vi "CRYDigital IO Setting.vi"(6 "No.VI":i32, 10 "Message Cluster":T1={"Name"="Default", "Type"=0, "Command Msg"="<Enter message or command here>", "Flags"=0, "Dialog?"=FALSE, "Numeric?"=FALSE, "Wait?"=FALSE, "Pause [ms]"=0, "pattern"=0, "Address"="", "Operation"=0, "bytes"=0, "Line selected"=0, "RS232 Func"=0, "Serial Ctrl lines"=0, "Interf #"=0, "GPIB func"=0, "GPIB cmd"=0, "GPIB rem en"=FALSE, "GPIB term"=0, "Curves generated"=[], "Units"={"unit"="", "dB ref"=0.0, "axis"=0, "data"=0, "Common dB ref."=1}, "Axis"=0, "Default Value"=0.0, "Message Tilte"="", "Port #"=0, "Print Unit"="", "Text Format"={"Size"=0, "Plain"=FALSE, "Bold"=FALSE, "Italic"=FALSE, "Underline"=FALSE, "Strikethrough"=FALSE, "Color"=0, "Font"=""}, "Help"="", "Tab Value"=enum."Setting", "pattern 2"=0, "Line selected 2"=0, "H_Bits"=[], "G_Bits"=[]} {"pattern 2" format="%.0b"; "Units"."Common dB ref." items=["dB", "dBSPL", "dBPa", "dBV", "dBm", "dBu", "dBFS"]; "Units"."dB ref" format="%.2f"; "pattern" format="%.0b"; "Flags" items=["Pass", "Fail"]}) -> (0 "Result":bool, 3 "Message Cluster Out":T1={"Name"="Default", "Type"=0, "Command Msg"="<Enter message or command here>", "Flags"=0, "Dialog?"=FALSE, "Numeric?"=FALSE, "Wait?"=FALSE, "Pause [ms]"=0, "pattern"=0, "Address"="", "Operation"=0, "bytes"=0, "Line selected"=0, "RS232 Func"=0, "Serial Ctrl lines"=0, "Interf #"=0, "GPIB func"=0, "GPIB cmd"=0, "GPIB rem en"=FALSE, "GPIB term"=0, "Curves generated"=[], "Units"={"unit"="", "dB ref"=0.0, "axis"=0, "data"=0, "Common dB ref."=1}, "Axis"=0, "Default Value"=0.0, "Message Tilte"="", "Port #"=0, "Print Unit"="", "Text Format"={"Size"=0, "Plain"=FALSE, "Bold"=FALSE, "Italic"=FALSE, "Underline"=FALSE, "Strikethrough"=FALSE, "Color"=0, "Font"=""}, "Help"="", "Tab Value"=enum."Setting", "pattern 2"=0, "Line selected 2"=0, "H_Bits"=[], "G_Bits"=[]} {"pattern 2" format="%.0b"; "Units"."Common dB ref." items=["dB", "dBSPL", "dBPa", "dBV", "dBm", "dBu", "dBFS"]; "Units"."dB ref" format="%.2f"; "pattern" format="%.0b"; "Flags" items=["Pass", "Fail"]})   [LabVIEW 2013]
uses:
  Typedef Control/CRYMessages Cluster.ctl
panel:
  out "H Selected":bool[](array[boolean])
  out "G Selected":bool[](array[boolean])
  out "Total_Comment":string
  out "True_Comment":string
  out "False_Comment":string
  out "G_Bits Out":T2(array[cluster])
  out "H_Bits Out":T2(array[cluster])
  out "Invert True":bool=TRUE caption="Invert"
  out "Invert False":bool=TRUE caption="Invert"
  in  "Setting Tab":enum32{"Port G", "Port H"}(tab)
  in  "G_Invert 2":bool=TRUE caption="Invert"
  in  "G_Invert 0":bool=TRUE caption="Invert"
  in  "G_Bit 4":i32[](listbox) caption="Bit 4"
  in  "G_Bit 0":i32[](listbox) caption="Bit 0"
  in  "G_Bit 1":i32[](listbox) caption="Bit 1"
  in  "G_Bit 3":i32[](listbox) caption="Bit 3"
  in  "G_Bit 5":i32[](listbox) caption="Bit 5"
  in  "G_Bit 7":i32[](listbox) caption="Bit 7"
  in  "G_Invert 1":bool=TRUE caption="Invert"
  in  "G_All 0":bool=TRUE caption="All"
  in  "G_All 1":bool=TRUE caption="All"
  in  "G_All 2":bool=TRUE caption="All"
  in  "G_All 3":bool=TRUE caption="All"
  in  "G_All 4":bool=TRUE caption="All"
  in  "G_All 5":bool=TRUE caption="All"
  in  "G_All 6":bool=TRUE caption="All"
  in  "G_All 7":bool=TRUE caption="All"
  in  "G_Invert 3":bool=TRUE caption="Invert"
  in  "G_Bit 2":i32[](listbox) caption="Bit 2"
  in  "G_Invert 4":bool=TRUE caption="Invert"
  in  "G_Invert 5":bool=TRUE caption="Invert"
  in  "G_Invert 6":bool=TRUE caption="Invert"
  in  "G_Bit 6":i32[](listbox) caption="Bit 6"
  in  "G_Invert 7":bool=TRUE caption="Invert"
  in  "H_All 0":bool=TRUE caption="All"
  in  "H_All 1":bool=TRUE caption="All"
  in  "H_All 2":bool=TRUE caption="All"
  in  "H_All 3":bool=TRUE caption="All"
  in  "H_All 4":bool=TRUE caption="All"
  in  "H_All 5":bool=TRUE caption="All"
  in  "H_All 6":bool=TRUE caption="All"
  in  "H_All 7":bool=TRUE caption="All"
  in  "H_Bit 7":i32[](listbox) caption="Bit 7"
  in  "H_Invert 7":bool=TRUE caption="Invert"
  in  "H_Bit 6":i32[](listbox) caption="Bit 6"
  in  "H_Invert 6":bool=TRUE caption="Invert"
  in  "H_Bit 5":i32[](listbox) caption="Bit 5"
  in  "H_Invert 5":bool=TRUE caption="Invert"
  in  "H_Bit 4":i32[](listbox) caption="Bit 4"
  in  "H_Invert 4":bool=TRUE caption="Invert"
  in  "H_Bit 3":i32[](listbox) caption="Bit 3"
  in  "H_Invert 3":bool=TRUE caption="Invert"
  in  "H_Bit 2":i32[](listbox) caption="Bit 2"
  in  "H_Invert 2":bool=TRUE caption="Invert"
  in  "H_Bit 1":i32[](listbox) caption="Bit 1"
  in  "H_Invert 1":bool=TRUE caption="Invert"
  in  "H_Bit 0":i32[](listbox) caption="Bit 0"
  in  "H_Invert 0":bool=TRUE caption="Invert"
  in  "Cancel":bool
  in  "OK":bool
  # "Ture = On     False = Off"
  # "Ture = Off     False = On"
  # "The results are \"Boolean And\" of items selected."
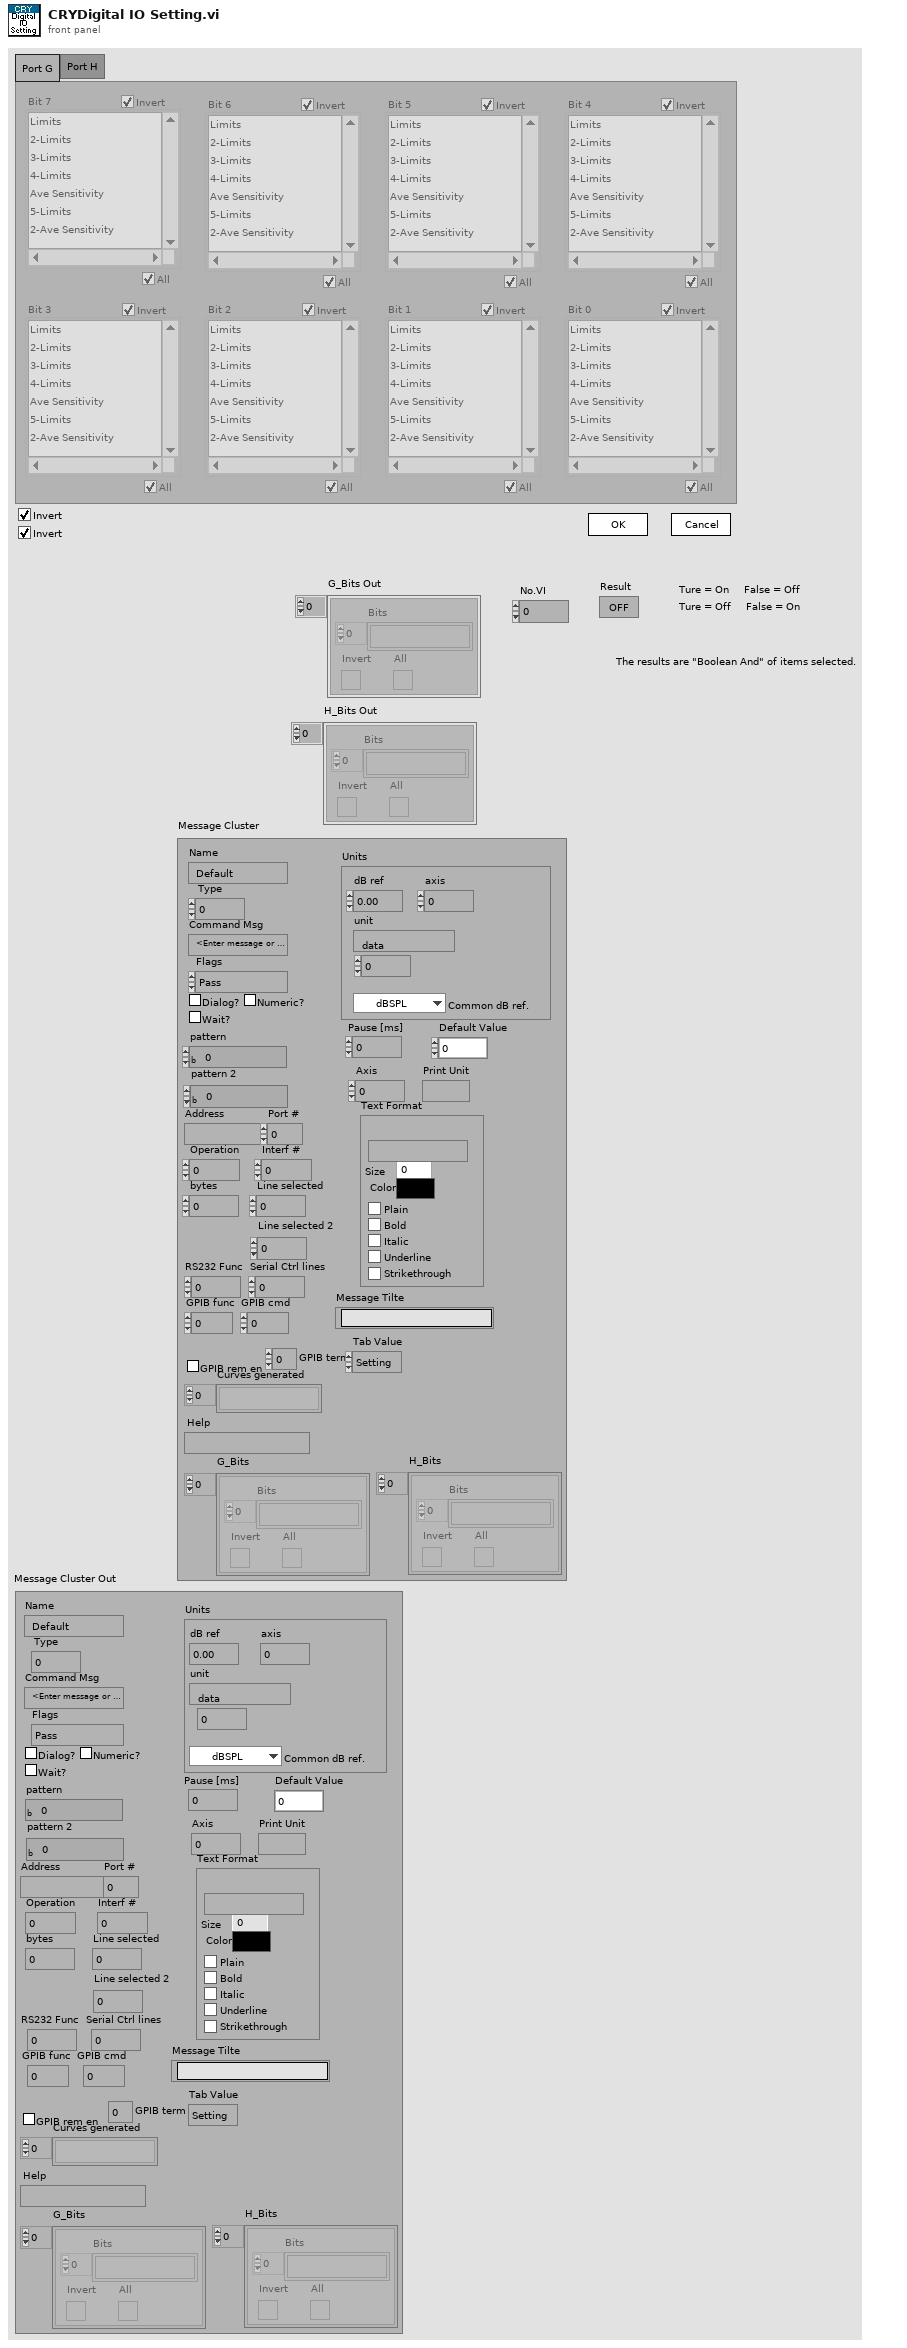
[diagram p1: front panel]
types:
  T1 = typedef "CRYMessages Cluster.ctl" = cluster{"Name":string, "Type":u16, "Command Msg":string, "Flags":u16, "Dialog?":bool, "Numeric?":bool, "Wait?":bool, "Pause [ms]":i32, "pattern":u32, "Address":string, "Operation":i32, "bytes":i32, "Line selected":u32, "RS232 Func":u16, "Serial Ctrl lines":u16, "Interf #":u8, "GPIB func":u16, "GPIB cmd":u16, "GPIB rem en":bool, "GPIB term":i32, "Curves generated":string[], "Units":cluster{"unit":string, "dB ref":dbl, "axis":u16, "data":u16, "Common dB ref.":u16}, "Axis":u16, "Default Value":dbl, "Message Tilte":string, "Port #":i32, "Print Unit":string, "Text Format":cluster{"Size":u32, "Plain":bool, "Bold":bool, "Italic":bool, "Underline":bool, "Strikethrough":bool, "Color":u32, "Font":string}, "Help":string, "Tab Value":enum32{"Setting", "Help"}, "pattern 2":u32, "Line selected 2":u32, "H_Bits":cluster{"Bits":string[], "Invert":bool, "All":bool}[], "G_Bits":cluster{"Bits":string[], "Invert":bool, "All":bool}[]}
  T2 = cluster{"Bits":string[], "Invert":bool, "All":bool}[]
  T3 = enum8{"Enabled", "Disabled", "Disabled and Grayed Out"}
  T4 = typedef "CRYResult Cluster Array.ctl" = T5[]
  T5 = typedef "CRYResult Cluster.ctl" = cluster{"Name":string, "Margin":dbl, "unit":string, "Verdict":bool, "Limit":string, "Max/Min":string, "protected":bool, "Step No.":i32, "Test Info":string, "AutoProtect":bool}
  T6 = cluster{"Bits":string[], "Invert":bool, "All":bool}
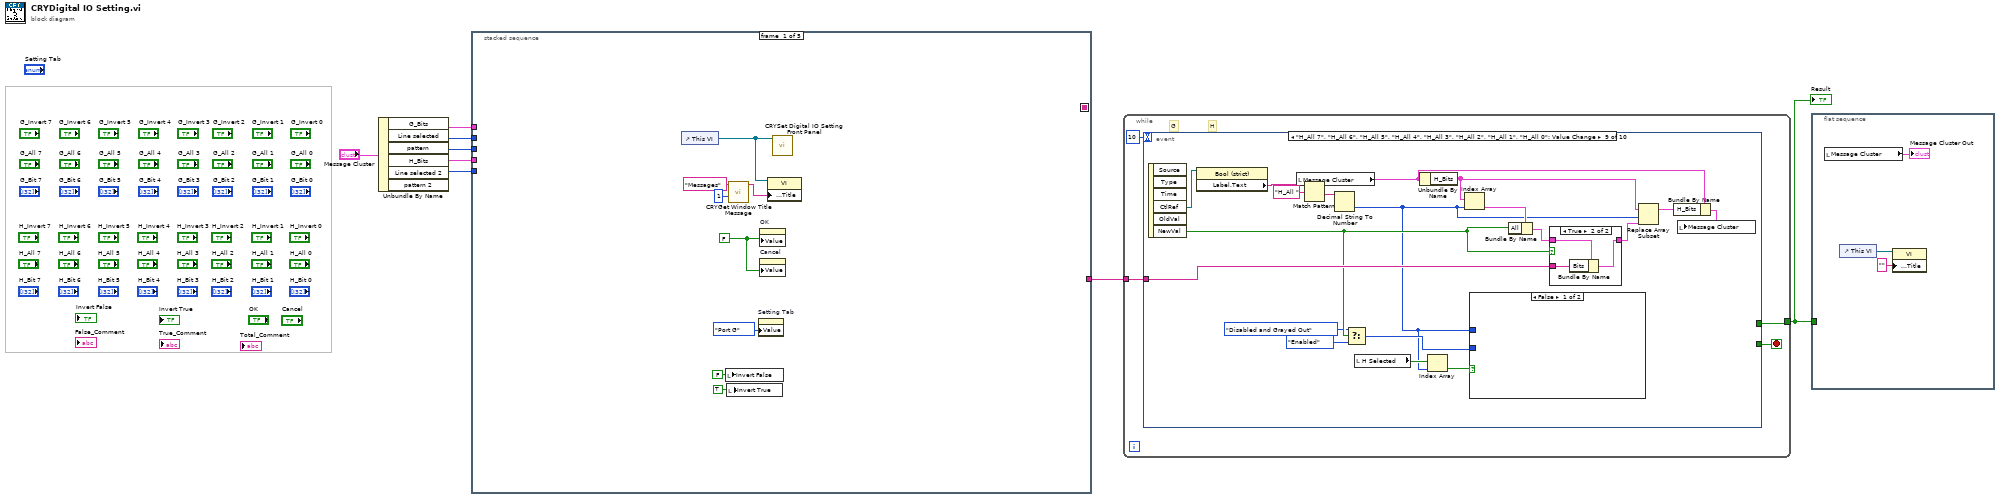
[diagram p0: block diagram]
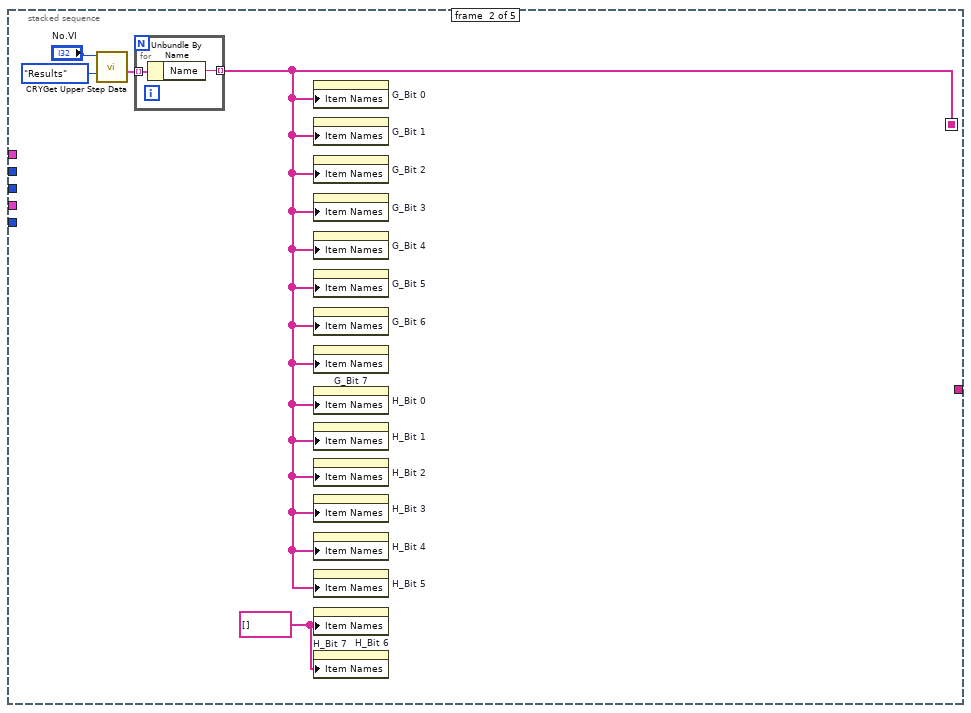
[diagram p2: hidden frame]
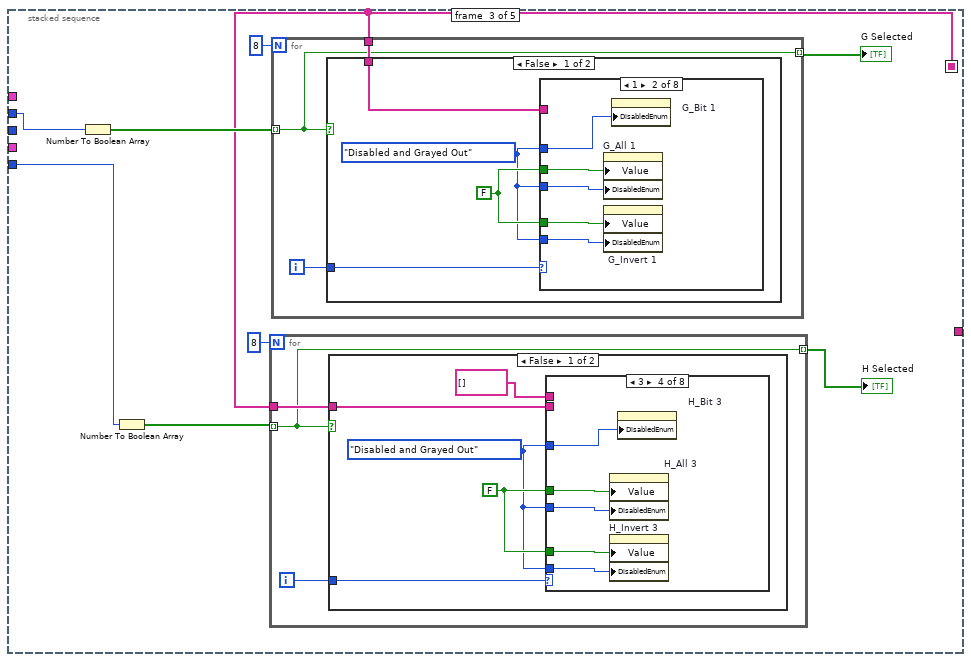
[diagram p3: hidden frame]
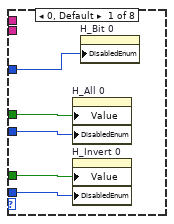
[diagram p4: hidden frame]
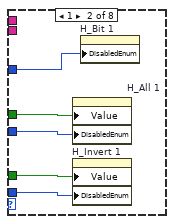
[diagram p5: hidden frame]
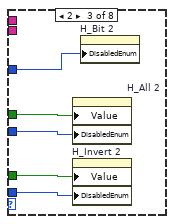
[diagram p6: hidden frame]
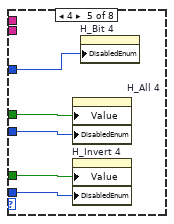
[diagram p7: hidden frame]
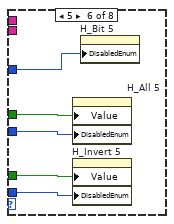
[diagram p8: hidden frame]
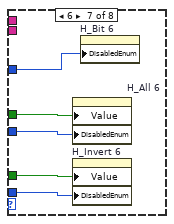
[diagram p9: hidden frame]
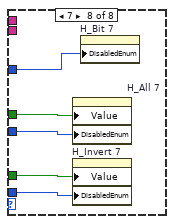
[diagram p10: hidden frame]
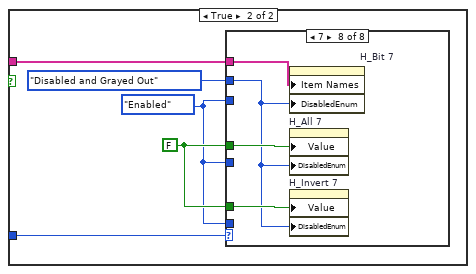
[diagram p11: hidden frame]
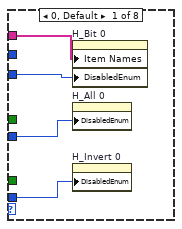
[diagram p12: hidden frame]
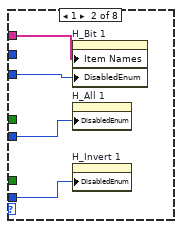
[diagram p13: hidden frame]
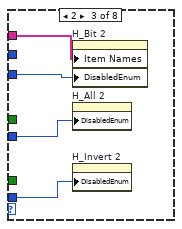
[diagram p14: hidden frame]
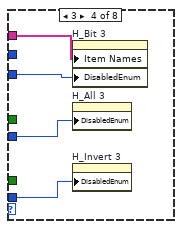
[diagram p15: hidden frame]
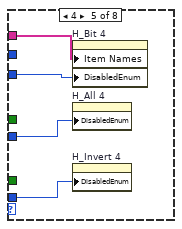
[diagram p16: hidden frame]
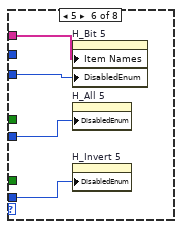
[diagram p17: hidden frame]
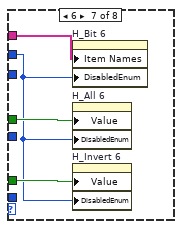
[diagram p18: hidden frame]
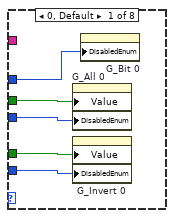
[diagram p19: hidden frame]
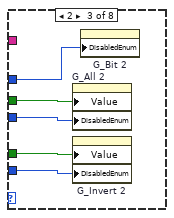
[diagram p20: hidden frame]
diagram:
  n1 = Unbundle By Name("Message Cluster") -> ("G_Bits"=w3:T2, "Line selected"=w6:u32, "pattern"=w1:u32, "H_Bits"=w4:T2, "Line selected 2"=w5:u32)  [unwired: 1 out]
  n2 = stacked-sequence {
    seq-local: [_ w18 _ _ _] -> [_ _ w27 w200 _]
    tunnel: [_ _ _ w200 _] -> w8
    tunnel: w3 -> [_ _ _ w199 _]
    tunnel: w4 -> [_ _ _ w198 _]
    tunnel: w6 -> [_ _ w32 w195 _]
    tunnel: w5 -> [_ _ w28 w193 _]
    tunnel: w1 -> [_ _ _ _ _]
    frame #0 {
      w16 = FALSE
      n3 = control-ref of="This VI"() -> (w13:refnum<vi>)
      n4 = local write "Invert False"(FALSE ("Invert False")) -> ()
      n5 = local write "Invert True"(TRUE ("Invert True")) -> ()
      n6 = call "CRYGet Window Title Message.vi"("No"=1, "Kind"="Messages") -> ("Multibyte String"=w12:string)  [unwired: 4 in, 5 out]
      n7 = property on="Setting Tab" class="TabCtl (strict)"("Value"=enum32{"Port G", "Port H"}."Port G" ("Setting Tab")) -> ()  [unwired: 2 in, 2 out]
      n8 = property on="OK" class="Bool (strict)"("Value"=w16) -> ()  [unwired: 2 in, 2 out]
      n9 = property on="Cancel" class="Bool (strict)"("Value"=w16) -> ()  [unwired: 2 in, 2 out]
      n10 = property class="VI"(reference=w13, "Front Panel.Title"=w12) -> ()  [unwired: 1 in, 2 out]
      n11 = call "CRYSet Digital IO Setting Front Panel.vi"("Vi Ref"=w13) -> ()  [unwired: 11 in]
    }
    frame #1 {
      w17 = string[] [] ("Item Names")
      n12 = call "CRYGet Upper Step Data.vi"("Type In"=enum16{"Curves", "Values", "Results", "WFM"}."Results", "No.VI"="No.VI") -> ("Result array"=w19:T4)  [unwired: 9 out]
      n13 = for {
        tunnel: w19 -> [w23] mode=indexing
        tunnel: [w22] -> w18 mode=indexing
        n14 = Unbundle By Name(w23) -> ("Name"=w22:string)
      }
      n15 = property on="G_Bit 0" class="LstBox (strict)"("Item Names"=w18) -> ()  [unwired: 2 in, 2 out]
      n16 = property on="G_Bit 1" class="LstBox (strict)"("Item Names"=w18) -> ()  [unwired: 2 in, 2 out]
      n17 = property on="G_Bit 2" class="LstBox (strict)"("Item Names"=w18) -> ()  [unwired: 2 in, 2 out]
      n18 = property on="G_Bit 3" class="LstBox (strict)"("Item Names"=w18) -> ()  [unwired: 2 in, 2 out]
      n19 = property on="G_Bit 4" class="LstBox (strict)"("Item Names"=w18) -> ()  [unwired: 2 in, 2 out]
      n20 = property on="G_Bit 5" class="LstBox (strict)"("Item Names"=w18) -> ()  [unwired: 2 in, 2 out]
      n21 = property on="G_Bit 6" class="LstBox (strict)"("Item Names"=w18) -> ()  [unwired: 2 in, 2 out]
      n22 = property on="G_Bit 7" class="LstBox (strict)"("Item Names"=w18) -> ()  [unwired: 2 in, 2 out]
      n23 = property on="H_Bit 0" class="LstBox (strict)"("Item Names"=w18) -> ()  [unwired: 2 in, 2 out]
      n24 = property on="H_Bit 1" class="LstBox (strict)"("Item Names"=w18) -> ()  [unwired: 2 in, 2 out]
      n25 = property on="H_Bit 2" class="LstBox (strict)"("Item Names"=w18) -> ()  [unwired: 2 in, 2 out]
      n26 = property on="H_Bit 3" class="LstBox (strict)"("Item Names"=w18) -> ()  [unwired: 2 in, 2 out]
      n27 = property on="H_Bit 4" class="LstBox (strict)"("Item Names"=w18) -> ()  [unwired: 2 in, 2 out]
      n28 = property on="H_Bit 5" class="LstBox (strict)"("Item Names"=w18) -> ()  [unwired: 2 in, 2 out]
      n29 = property on="H_Bit 6" class="LstBox (strict)"("Item Names"=w17) -> ()  [unwired: 2 in, 2 out]
      n30 = property on="H_Bit 7" class="LstBox (strict)"("Item Names"=w17) -> ()  [unwired: 2 in, 2 out]
    }
    frame #2 {
      n31 = Number To Boolean Array(number=w32) -> (Boolean array=w31:bool[])
      n32 = Number To Boolean Array(number=w28) -> (Boolean array=w29:bool[])
      n33 = for {
        N: 8 -> [_]
        tunnel: w29 -> [w33] mode=indexing
        tunnel: w27 -> [w34]
        tunnel: [w33] -> w24 mode=indexing
        i -> [w35]
        n34 = case shown="False" w33 {
          tunnel: w35 -> [w40 w85]
          tunnel: w34 -> [w37 w82]
          frame False {
            w39 = FALSE ("H_All 0")
            w38 = T3."Disabled and Grayed Out" ("Disabled")
            n35 = case shown="3" w40 {
              tunnel: w38 -> [w45 w50 w55 w60 w65 w70 w75 w80]
              tunnel: w39 -> [w44 w49 w54 w59 w64 w69 w74 w79]
              tunnel: w38 -> [w43 w48 w53 w58 w63 w68 w73 w78]
              tunnel: w39 -> [w42 w47 w52 w57 w62 w67 w72 w77]
              tunnel: w38 -> [w41 w46 w51 w56 w61 w66 w71 w76]
              tunnel: w37 -> [_ _ _ _ _ _ _ _]
              tunnel: string[] [] ("Item Names") -> [_ _ _ _ _ _ _ _]
              frame 0, Default {
                n36 = property on="H_All 0" class="Bool (strict)"("Value"=w44, "DisabledEnum"=w43) -> ()  [unwired: 2 in, 2 out]
                n37 = property on="H_Invert 0" class="Bool (strict)"("Value"=w42, "DisabledEnum"=w41) -> ()  [unwired: 2 in, 2 out]
                n38 = property on="H_Bit 0" class="LstBox (strict)"("DisabledEnum"=w45) -> ()  [unwired: 2 in, 2 out]
              }
              frame 1 {
                n39 = property on="H_All 1" class="Bool (strict)"("Value"=w49, "DisabledEnum"=w48) -> ()  [unwired: 2 in, 2 out]
                n40 = property on="H_Invert 1" class="Bool (strict)"("Value"=w47, "DisabledEnum"=w46) -> ()  [unwired: 2 in, 2 out]
                n41 = property on="H_Bit 1" class="LstBox (strict)"("DisabledEnum"=w50) -> ()  [unwired: 2 in, 2 out]
              }
              frame 2 {
                n42 = property on="H_All 2" class="Bool (strict)"("Value"=w54, "DisabledEnum"=w53) -> ()  [unwired: 2 in, 2 out]
                n43 = property on="H_Invert 2" class="Bool (strict)"("Value"=w52, "DisabledEnum"=w51) -> ()  [unwired: 2 in, 2 out]
                n44 = property on="H_Bit 2" class="LstBox (strict)"("DisabledEnum"=w55) -> ()  [unwired: 2 in, 2 out]
              }
              frame 3 {
                n45 = property on="H_All 3" class="Bool (strict)"("Value"=w59, "DisabledEnum"=w58) -> ()  [unwired: 2 in, 2 out]
                n46 = property on="H_Invert 3" class="Bool (strict)"("Value"=w57, "DisabledEnum"=w56) -> ()  [unwired: 2 in, 2 out]
                n47 = property on="H_Bit 3" class="LstBox (strict)"("DisabledEnum"=w60) -> ()  [unwired: 2 in, 2 out]
              }
              frame 4 {
                n48 = property on="H_All 4" class="Bool (strict)"("Value"=w64, "DisabledEnum"=w63) -> ()  [unwired: 2 in, 2 out]
                n49 = property on="H_Invert 4" class="Bool (strict)"("Value"=w62, "DisabledEnum"=w61) -> ()  [unwired: 2 in, 2 out]
                n50 = property on="H_Bit 4" class="LstBox (strict)"("DisabledEnum"=w65) -> ()  [unwired: 2 in, 2 out]
              }
              frame 5 {
                n51 = property on="H_All 5" class="Bool (strict)"("Value"=w69, "DisabledEnum"=w68) -> ()  [unwired: 2 in, 2 out]
                n52 = property on="H_Invert 5" class="Bool (strict)"("Value"=w67, "DisabledEnum"=w66) -> ()  [unwired: 2 in, 2 out]
                n53 = property on="H_Bit 5" class="LstBox (strict)"("DisabledEnum"=w70) -> ()  [unwired: 2 in, 2 out]
              }
              frame 6 {
                n54 = property on="H_All 6" class="Bool (strict)"("Value"=w74, "DisabledEnum"=w73) -> ()  [unwired: 2 in, 2 out]
                n55 = property on="H_Invert 6" class="Bool (strict)"("Value"=w72, "DisabledEnum"=w71) -> ()  [unwired: 2 in, 2 out]
                n56 = property on="H_Bit 6" class="LstBox (strict)"("DisabledEnum"=w75) -> ()  [unwired: 2 in, 2 out]
              }
              frame 7 {
                n57 = property on="H_All 7" class="Bool (strict)"("Value"=w79, "DisabledEnum"=w78) -> ()  [unwired: 2 in, 2 out]
                n58 = property on="H_Invert 7" class="Bool (strict)"("Value"=w77, "DisabledEnum"=w76) -> ()  [unwired: 2 in, 2 out]
                n59 = property on="H_Bit 7" class="LstBox (strict)"("DisabledEnum"=w80) -> ()  [unwired: 2 in, 2 out]
              }
            }
          }
          frame True {
            w84 = FALSE ("H_All 0")
            w83 = T3."Enabled" ("Disabled")
            n60 = case shown="7" w85 {
              tunnel: w83 -> [w89 w93 w97 w101 w105 w109 _ _]
              tunnel: w84 -> [_ _ _ _ _ _ w113 w117]
              tunnel: w83 -> [w88 w92 w96 w100 w104 w108 _ _]
              tunnel: w84 -> [_ _ _ _ _ _ w112 w116]
              tunnel: w83 -> [w87 w91 w95 w99 w103 w107 _ _]
              tunnel: w82 -> [w86 w90 w94 w98 w102 w106 w111 w115]
              tunnel: T3."Disabled and Grayed Out" ("Disabled") -> [_ _ _ _ _ _ w110 w114]
              frame 0, Default {
                n61 = property on="H_Bit 0" class="LstBox (strict)"("Item Names"=w86, "DisabledEnum"=w89) -> ()  [unwired: 2 in, 2 out]
                n62 = property on="H_All 0" class="Bool (strict)"("DisabledEnum"=w88) -> ()  [unwired: 2 in, 2 out]
                n63 = property on="H_Invert 0" class="Bool (strict)"("DisabledEnum"=w87) -> ()  [unwired: 2 in, 2 out]
              }
              frame 1 {
                n64 = property on="H_Bit 1" class="LstBox (strict)"("Item Names"=w90, "DisabledEnum"=w93) -> ()  [unwired: 2 in, 2 out]
                n65 = property on="H_All 1" class="Bool (strict)"("DisabledEnum"=w92) -> ()  [unwired: 2 in, 2 out]
                n66 = property on="H_Invert 1" class="Bool (strict)"("DisabledEnum"=w91) -> ()  [unwired: 2 in, 2 out]
              }
              frame 2 {
                n67 = property on="H_Bit 2" class="LstBox (strict)"("Item Names"=w94, "DisabledEnum"=w97) -> ()  [unwired: 2 in, 2 out]
                n68 = property on="H_All 2" class="Bool (strict)"("DisabledEnum"=w96) -> ()  [unwired: 2 in, 2 out]
                n69 = property on="H_Invert 2" class="Bool (strict)"("DisabledEnum"=w95) -> ()  [unwired: 2 in, 2 out]
              }
              frame 3 {
                n70 = property on="H_Bit 3" class="LstBox (strict)"("Item Names"=w98, "DisabledEnum"=w101) -> ()  [unwired: 2 in, 2 out]
                n71 = property on="H_All 3" class="Bool (strict)"("DisabledEnum"=w100) -> ()  [unwired: 2 in, 2 out]
                n72 = property on="H_Invert 3" class="Bool (strict)"("DisabledEnum"=w99) -> ()  [unwired: 2 in, 2 out]
              }
              frame 4 {
                n73 = property on="H_Bit 4" class="LstBox (strict)"("Item Names"=w102, "DisabledEnum"=w105) -> ()  [unwired: 2 in, 2 out]
                n74 = property on="H_All 4" class="Bool (strict)"("DisabledEnum"=w104) -> ()  [unwired: 2 in, 2 out]
                n75 = property on="H_Invert 4" class="Bool (strict)"("DisabledEnum"=w103) -> ()  [unwired: 2 in, 2 out]
              }
              frame 5 {
                n76 = property on="H_Bit 5" class="LstBox (strict)"("Item Names"=w106, "DisabledEnum"=w109) -> ()  [unwired: 2 in, 2 out]
                n77 = property on="H_All 5" class="Bool (strict)"("DisabledEnum"=w108) -> ()  [unwired: 2 in, 2 out]
                n78 = property on="H_Invert 5" class="Bool (strict)"("DisabledEnum"=w107) -> ()  [unwired: 2 in, 2 out]
              }
              frame 6 {
                n79 = property on="H_Bit 6" class="LstBox (strict)"("Item Names"=w111, "DisabledEnum"=w110) -> ()  [unwired: 2 in, 2 out]
                n80 = property on="H_All 6" class="Bool (strict)"("Value"=w113, "DisabledEnum"=w110) -> ()  [unwired: 2 in, 2 out]
                n81 = property on="H_Invert 6" class="Bool (strict)"("Value"=w112, "DisabledEnum"=w110) -> ()  [unwired: 2 in, 2 out]
              }
              frame 7 {
                n82 = property on="H_Bit 7" class="LstBox (strict)"("Item Names"=w115, "DisabledEnum"=w114) -> ()  [unwired: 2 in, 2 out]
                n83 = property on="H_All 7" class="Bool (strict)"("Value"=w117, "DisabledEnum"=w114) -> ()  [unwired: 2 in, 2 out]
                n84 = property on="H_Invert 7" class="Bool (strict)"("Value"=w116, "DisabledEnum"=w114) -> ()  [unwired: 2 in, 2 out]
              }
            }
          }
        }
      }
      "H Selected" <- w24
      n85 = for {
        N: 8 -> [_]
        tunnel: w31 -> [w118] mode=indexing
        tunnel: w27 -> [w119]
        tunnel: [w118] -> w25 mode=indexing
        i -> [w120]
        n86 = case shown="False" w118 {
          tunnel: w120 -> [w124 w167]
          tunnel: w119 -> [w121 w165]
          frame False {
            w123 = FALSE ("H_All 0")
            w122 = T3."Disabled and Grayed Out" ("Disabled")
            n87 = case shown="1" w124 {
              tunnel: w122 -> [w129 w134 w139 w144 w149 w154 w159 w164]
              tunnel: w123 -> [w128 w133 w138 w143 w148 w153 w158 w163]
              tunnel: w122 -> [w127 w132 w137 w142 w147 w152 w157 w162]
              tunnel: w123 -> [w126 w131 w136 w141 w146 w151 w156 w161]
              tunnel: w122 -> [w125 w130 w135 w140 w145 w150 w155 w160]
              tunnel: w121 -> [_ _ _ _ _ _ _ _]
              frame 0, Default {
                n88 = property on="G_All 0" class="Bool (strict)"("Value"=w128, "DisabledEnum"=w127) -> ()  [unwired: 2 in, 2 out]
                n89 = property on="G_Invert 0" class="Bool (strict)"("Value"=w126, "DisabledEnum"=w125) -> ()  [unwired: 2 in, 2 out]
                n90 = property on="G_Bit 0" class="LstBox (strict)"("DisabledEnum"=w129) -> ()  [unwired: 2 in, 2 out]
              }
              frame 1 {
                n91 = property on="G_All 1" class="Bool (strict)"("Value"=w133, "DisabledEnum"=w132) -> ()  [unwired: 2 in, 2 out]
                n92 = property on="G_Invert 1" class="Bool (strict)"("Value"=w131, "DisabledEnum"=w130) -> ()  [unwired: 2 in, 2 out]
                n93 = property on="G_Bit 1" class="LstBox (strict)"("DisabledEnum"=w134) -> ()  [unwired: 2 in, 2 out]
              }
              frame 2 {
                n94 = property on="G_All 2" class="Bool (strict)"("Value"=w138, "DisabledEnum"=w137) -> ()  [unwired: 2 in, 2 out]
                n95 = property on="G_Invert 2" class="Bool (strict)"("Value"=w136, "DisabledEnum"=w135) -> ()  [unwired: 2 in, 2 out]
                n96 = property on="G_Bit 2" class="LstBox (strict)"("DisabledEnum"=w139) -> ()  [unwired: 2 in, 2 out]
              }
              frame 3 {
                n97 = property on="G_All 3" class="Bool (strict)"("Value"=w143, "DisabledEnum"=w142) -> ()  [unwired: 2 in, 2 out]
                n98 = property on="G_Invert 3" class="Bool (strict)"("Value"=w141, "DisabledEnum"=w140) -> ()  [unwired: 2 in, 2 out]
                n99 = property on="G_Bit 3" class="LstBox (strict)"("DisabledEnum"=w144) -> ()  [unwired: 2 in, 2 out]
              }
              frame 4 {
                n100 = property on="G_All 4" class="Bool (strict)"("Value"=w148, "DisabledEnum"=w147) -> ()  [unwired: 2 in, 2 out]
                n101 = property on="G_Invert 4" class="Bool (strict)"("Value"=w146, "DisabledEnum"=w145) -> ()  [unwired: 2 in, 2 out]
                n102 = property on="G_Bit 4" class="LstBox (strict)"("DisabledEnum"=w149) -> ()  [unwired: 2 in, 2 out]
              }
              frame 5 {
                n103 = property on="G_All 5" class="Bool (strict)"("Value"=w153, "DisabledEnum"=w152) -> ()  [unwired: 2 in, 2 out]
                n104 = property on="G_Invert 5" class="Bool (strict)"("Value"=w151, "DisabledEnum"=w150) -> ()  [unwired: 2 in, 2 out]
                n105 = property on="G_Bit 5" class="LstBox (strict)"("DisabledEnum"=w154) -> ()  [unwired: 2 in, 2 out]
              }
              frame 6 {
                n106 = property on="G_All 6" class="Bool (strict)"("Value"=w158, "DisabledEnum"=w157) -> ()  [unwired: 2 in, 2 out]
                n107 = property on="G_Invert 6" class="Bool (strict)"("Value"=w156, "DisabledEnum"=w155) -> ()  [unwired: 2 in, 2 out]
                n108 = property on="G_Bit 6" class="LstBox (strict)"("DisabledEnum"=w159) -> ()  [unwired: 2 in, 2 out]
              }
              frame 7 {
                n109 = property on="G_All 7" class="Bool (strict)"("Value"=w163, "DisabledEnum"=w162) -> ()  [unwired: 2 in, 2 out]
                n110 = property on="G_Invert 7" class="Bool (strict)"("Value"=w161, "DisabledEnum"=w160) -> ()  [unwired: 2 in, 2 out]
                n111 = property on="G_Bit 7" class="LstBox (strict)"("DisabledEnum"=w164) -> ()  [unwired: 2 in, 2 out]
              }
            }
          }
          frame True {
            w166 = T3."Enabled" ("Disabled")
            n112 = case shown="0, Default" w167 {
              tunnel: w166 -> [w170 w173 w176 w179 w182 w185 w188 w191]
              tunnel: w166 -> [w169 w172 w175 w178 w181 w184 w187 w190]
              tunnel: w166 -> [w168 w171 w174 w177 w180 w183 w186 w189]
              tunnel: w165 -> [_ _ _ _ _ _ _ _]
              frame 0, Default {
                n113 = property on="G_All 0" class="Bool (strict)"("DisabledEnum"=w169) -> ()  [unwired: 2 in, 2 out]
                n114 = property on="G_Invert 0" class="Bool (strict)"("DisabledEnum"=w168) -> ()  [unwired: 2 in, 2 out]
                n115 = property on="G_Bit 0" class="LstBox (strict)"("DisabledEnum"=w170) -> ()  [unwired: 2 in, 2 out]
              }
              frame 1 {
                n116 = property on="G_All 1" class="Bool (strict)"("DisabledEnum"=w172) -> ()  [unwired: 2 in, 2 out]
                n117 = property on="G_Invert 1" class="Bool (strict)"("DisabledEnum"=w171) -> ()  [unwired: 2 in, 2 out]
                n118 = property on="G_Bit 1" class="LstBox (strict)"("DisabledEnum"=w173) -> ()  [unwired: 2 in, 2 out]
              }
              frame 2 {
                n119 = property on="G_All 2" class="Bool (strict)"("DisabledEnum"=w175) -> ()  [unwired: 2 in, 2 out]
                n120 = property on="G_Invert 2" class="Bool (strict)"("DisabledEnum"=w174) -> ()  [unwired: 2 in, 2 out]
                n121 = property on="G_Bit 2" class="LstBox (strict)"("DisabledEnum"=w176) -> ()  [unwired: 2 in, 2 out]
              }
              frame 3 {
                n122 = property on="G_All 3" class="Bool (strict)"("DisabledEnum"=w178) -> ()  [unwired: 2 in, 2 out]
                n123 = property on="G_Invert 3" class="Bool (strict)"("DisabledEnum"=w177) -> ()  [unwired: 2 in, 2 out]
                n124 = property on="G_Bit 3" class="LstBox (strict)"("DisabledEnum"=w179) -> ()  [unwired: 2 in, 2 out]
              }
              frame 4 {
                n125 = property on="G_All 4" class="Bool (strict)"("DisabledEnum"=w181) -> ()  [unwired: 2 in, 2 out]
                n126 = property on="G_Invert 4" class="Bool (strict)"("DisabledEnum"=w180) -> ()  [unwired: 2 in, 2 out]
                n127 = property on="G_Bit 4" class="LstBox (strict)"("DisabledEnum"=w182) -> ()  [unwired: 2 in, 2 out]
              }
              frame 5 {
                n128 = property on="G_All 5" class="Bool (strict)"("DisabledEnum"=w184) -> ()  [unwired: 2 in, 2 out]
                n129 = property on="G_Invert 5" class="Bool (strict)"("DisabledEnum"=w183) -> ()  [unwired: 2 in, 2 out]
                n130 = property on="G_Bit 5" class="LstBox (strict)"("DisabledEnum"=w185) -> ()  [unwired: 2 in, 2 out]
              }
              frame 6 {
                n131 = property on="G_All 6" class="Bool (strict)"("DisabledEnum"=w187) -> ()  [unwired: 2 in, 2 out]
                n132 = property on="G_Invert 6" class="Bool (strict)"("DisabledEnum"=w186) -> ()  [unwired: 2 in, 2 out]
                n133 = property on="G_Bit 6" class="LstBox (strict)"("DisabledEnum"=w188) -> ()  [unwired: 2 in, 2 out]
              }
              frame 7 {
                n134 = property on="G_All 7" class="Bool (strict)"("DisabledEnum"=w190) -> ()  [unwired: 2 in, 2 out]
                n135 = property on="G_Invert 7" class="Bool (strict)"("DisabledEnum"=w189) -> ()  [unwired: 2 in, 2 out]
                n136 = property on="G_Bit 7" class="LstBox (strict)"("DisabledEnum"=w191) -> ()  [unwired: 2 in, 2 out]
              }
            }
          }
        }
      }
      "G Selected" <- w25
    }
    frame #3 {
      n137 = Number To Boolean Array(number=w193) -> (Boolean array=w192:bool[])
      n138 = Number To Boolean Array(number=w195) -> (Boolean array=w194:bool[])
      n139 = control-ref of="This VI"() -> (w196:refnum<vi>)
      n140 = control-ref of="This VI"() -> (w197:refnum<vi>)
      n141 = for {
        tunnel: w199 -> [w243] mode=indexing
        tunnel: w197 -> [w242]
        tunnel: w200 -> [w240]
        tunnel: w194 -> [w239] mode=indexing
        i -> [w241]
        n142 = case shown="False" w239 {
          tunnel: w243 -> [_ w267]
          tunnel: w242 -> [w244 w266]
          tunnel: w241 -> [w245 w257]
          tunnel: w240 -> [_ w255]
          frame False {
            n143 = disable-structure shown="Disabled" {
              disable-tunnel: w245 -> [w251 _]
              disable-tunnel: w244 -> [w247 _]
              frame Disabled {
                n144 = Number To Decimal String(number=w251) -> (decimal integer string=w248:string)  [unwired: 1 in]
                n145 = Concatenate Strings("G_Bit " ("string"), w248) -> (w249:string)
                n146 = invoke class="VI" method="Ctrl Val.Set"(reference=w247, "Control Name"=w249, "Value"=i32[] []) -> ()  [unwired: 2 in, 5 out]
              }
              frame Enabled {
              }
            }
          }
          frame True {
            n147 = Unbundle By Name(w267) -> ("Bits"=w254:string[], "Invert"=w258:bool, "All"=w256:bool)
            n148 = Number To Decimal String(number=w257) -> (decimal integer string=w261:string)  [unwired: 1 in]
            n149 = for {
              tunnel: w255 -> [w271]
              tunnel: w254 -> [w272] mode=indexing
              shift-right: [w268] -> w252
              shift-left: i32[] [] -> [w269]
              n150 = Search 1D Array(1D array=w271, element=w272) -> (index of element=w270:i32)  [unwired: 1 in]
              n151 = case shown="-1" w270 {
                selector: w270 -> [w273 _]
                tunnel: w269 -> [w275 w276]
                tunnel: [w274 w276] -> w268
                frame 0, Default {
                  n152 = Insert Into Array(array=w275, new element=w273) -> (w274:i32[])  [unwired: 1 in]
                }
                frame -1 {
                }
              }
            }
            n153 = Concatenate Strings("G_Bit " ("string"), w261) -> (w264:string)
            n154 = Concatenate Strings("G_Invert " ("string"), w261) -> (w260:string)
            n155 = Concatenate Strings("G_All " ("string"), w261) -> (w259:string)
            n156 = invoke class="VI" method="Ctrl Val.Set"(reference=w266, "Control Name"=w264, "Value"=w252) -> ()  [unwired: 2 in, 5 out]
            n157 = invoke class="VI" method="Ctrl Val.Set"(reference=w266, "Control Name"=w260, "Value"=w258) -> ()  [unwired: 2 in, 5 out]
            n158 = invoke class="VI" method="Ctrl Val.Set"(reference=w266, "Control Name"=w259, "Value"=w256) -> ()  [unwired: 2 in, 5 out]
          }
        }
      }
      n159 = for {
        tunnel: w198 -> [w205] mode=indexing
        tunnel: w196 -> [w204]
        tunnel: w200 -> [w202]
        tunnel: w192 -> [w201] mode=indexing
        i -> [w203]
        n160 = case shown="False" w201 {
          tunnel: w205 -> [_ w229]
          tunnel: w204 -> [w206 w228]
          tunnel: w203 -> [w207 w219]
          tunnel: w202 -> [_ w217]
          frame False {
            n161 = disable-structure shown="Disabled" {
              disable-tunnel: w207 -> [w209 _]
              disable-tunnel: w206 -> [w208 _]
              frame Disabled {
                n162 = Number To Decimal String(number=w209) -> (decimal integer string=w212:string)  [unwired: 1 in]
                n163 = Concatenate Strings("H_Bit " ("string"), w212) -> (w211:string)
                n164 = invoke class="VI" method="Ctrl Val.Set"(reference=w208, "Control Name"=w211, "Value"=i32[] []) -> ()  [unwired: 2 in, 5 out]
              }
              frame Enabled {
              }
            }
          }
          frame True {
            n165 = Unbundle By Name(w229) -> ("Bits"=w216:string[], "Invert"=w220:bool, "All"=w218:bool)
            n166 = Number To Decimal String(number=w219) -> (decimal integer string=w223:string)  [unwired: 1 in]
            n167 = for {
              tunnel: w217 -> [w233]
              tunnel: w216 -> [w234] mode=indexing
              shift-right: [w230] -> w214
              shift-left: i32[] [] -> [w231]
              n168 = Search 1D Array(1D array=w233, element=w234) -> (index of element=w232:i32)  [unwired: 1 in]
              n169 = case shown="0, Default" w232 {
                selector: w232 -> [w235 _]
                tunnel: w231 -> [w237 w238]
                tunnel: [w236 w238] -> w230
                frame 0, Default {
                  n170 = Insert Into Array(array=w237, new element=w235) -> (w236:i32[])  [unwired: 1 in]
                }
                frame -1 {
                }
              }
            }
            n171 = Concatenate Strings("H_Bit " ("string"), w223) -> (w226:string)
            n172 = Concatenate Strings("H_Invert " ("string"), w223) -> (w222:string)
            n173 = Concatenate Strings("H_All " ("string"), w223) -> (w221:string)
            n174 = invoke class="VI" method="Ctrl Val.Set"(reference=w228, "Control Name"=w226, "Value"=w214) -> ()  [unwired: 2 in, 5 out]
            n175 = invoke class="VI" method="Ctrl Val.Set"(reference=w228, "Control Name"=w222, "Value"=w220) -> ()  [unwired: 2 in, 5 out]
            n176 = invoke class="VI" method="Ctrl Val.Set"(reference=w228, "Control Name"=w221, "Value"=w218) -> ()  [unwired: 2 in, 5 out]
          }
        }
      }
    }
    frame #4 {
      n177 = control-ref of="This VI"() -> (w296:refnum<vi>)
      n178 = for {
        N: 8 -> [_]
        tunnel: w296 -> [w303]
        tunnel: [w300] -> w295 mode=indexing
        tunnel: [w297] -> w286 mode=indexing
        i -> [w304]
        n179 = Number To Decimal String(number=w304) -> (decimal integer string=w310:string)  [unwired: 1 in]
        n180 = Number To Decimal String(number=w304) -> (decimal integer string=w307:string)  [unwired: 1 in]
        n181 = Concatenate Strings("H_All " ("string"), w307) -> (w305:string)
        n182 = Concatenate Strings("G_All " ("string"), w310) -> (w308:string)
        n183 = invoke class="VI" method="Ctrl Val.Get"(reference=w303, "Control Name"=w308) -> ("Get Control Value Variant"=w302:variant)  [unwired: 2 in, 3 out]
        n184 = invoke class="VI" method="Ctrl Val.Get"(reference=w303, "Control Name"=w305) -> ("Get Control Value Variant"=w299:variant)  [unwired: 2 in, 3 out]
        n185 = Variant To Data(type=FALSE ("Value (Signaling)"), Variant=w302) -> (data=w300:bool)  [unwired: 1 in, 1 out]
        n186 = Variant To Data(type=FALSE ("Value (Signaling)"), Variant=w299) -> (data=w297:bool)  [unwired: 1 in, 1 out]
      }
      n187 = Index Array(array=w295) -> (element #1=w294:bool, element #2=w293:bool, element #3=w292:bool, element #4=w291:bool, element #5=w290:bool, element #6=w289:bool, element #7=w288:bool, element #8=w287:bool)  [unwired: 8 in]
      n188 = Index Array(array=w286) -> (element #1=w285:bool, element #2=w284:bool, element #3=w283:bool, element #4=w282:bool, element #5=w281:bool, element #6=w280:bool, element #7=w278:bool, element #8=w279:bool)  [unwired: 8 in]
      n189 = property on="G_All 0" class="Bool (strict)"("Val(Sgnl)"=w294) -> ()  [unwired: 2 in, 2 out]
      n190 = property on="G_All 1" class="Bool (strict)"("Val(Sgnl)"=w293) -> ()  [unwired: 2 in, 2 out]
      n191 = property on="G_All 2" class="Bool (strict)"("Val(Sgnl)"=w292) -> ()  [unwired: 2 in, 2 out]
      n192 = property on="G_All 3" class="Bool (strict)"("Val(Sgnl)"=w291) -> ()  [unwired: 2 in, 2 out]
      n193 = property on="G_All 4" class="Bool (strict)"("Val(Sgnl)"=w290) -> ()  [unwired: 2 in, 2 out]
      n194 = property on="G_All 5" class="Bool (strict)"("Val(Sgnl)"=w289) -> ()  [unwired: 2 in, 2 out]
      n195 = property on="G_All 6" class="Bool (strict)"("Val(Sgnl)"=w288) -> ()  [unwired: 2 in, 2 out]
      n196 = property on="G_All 7" class="Bool (strict)"("Val(Sgnl)"=w287) -> ()  [unwired: 2 in, 2 out]
      n197 = property on="H_All 0" class="Bool (strict)"("Val(Sgnl)"=w285) -> ()  [unwired: 2 in, 2 out]
      n198 = property on="H_All 1" class="Bool (strict)"("Val(Sgnl)"=w284) -> ()  [unwired: 2 in, 2 out]
      n199 = property on="H_All 2" class="Bool (strict)"("Val(Sgnl)"=w283) -> ()  [unwired: 2 in, 2 out]
      n200 = property on="H_All 3" class="Bool (strict)"("Val(Sgnl)"=w282) -> ()  [unwired: 2 in, 2 out]
      n201 = property on="H_All 4" class="Bool (strict)"("Val(Sgnl)"=w281) -> ()  [unwired: 2 in, 2 out]
      n202 = property on="H_All 5" class="Bool (strict)"("Val(Sgnl)"=w280) -> ()  [unwired: 2 in, 2 out]
      n203 = property on="H_All 6" class="Bool (strict)"("Val(Sgnl)"=w278) -> ()  [unwired: 2 in, 2 out]
      n204 = property on="H_All 7" class="Bool (strict)"("Val(Sgnl)"=w279) -> ()  [unwired: 2 in, 2 out]
    }
  }
  n205 = while {
    tunnel: [w311] -> w7
    tunnel: w8 -> [w312]
    stop <- w313 stop-if-true
    # "G"
    # "H"
    n206 = event shown="[8] \"H_All 7\", \"H_All 6\", \"H_All 5\", \"H_All 4\", \"H_All 3\", \"H_All 2\", \"H_All 1\", \"H_All 0\": Value Change" {
      selector: _ -> [_ _ _ _ _ _ _ _ _ _]
      dyn-events: _ -> [_ _ _ _ _ _ _ _ _ _]
      timeout: 10 -> [_ _ _ _ _ _ _ _ _ _]
      tunnel: [_ w315 w319 TRUE ("NewVal") _ _ _ _ _ _] -> w313
      tunnel: w312 -> [_ _ _ _ _ _ _ _ w391 w428]
      tunnel: [_ w315 w318 FALSE ("NewVal") _ _ _ _ _ _] -> w311
      event Timeout {
        n207 = event-data() -> ()  [unwired: 3 out]
      }
      event "OK": Value Change {
        n208 = event-data() -> ("NewVal"=w315:bool)  [unwired: 6 out]
        n209 = disable-structure shown="Disabled" {
          frame Disabled {
            n210 = local read item#-1() -> (→"H_Bits Out")
            n211 = local read item#-1() -> (→"G_Bits Out")
          }
          frame Enabled {
          }
        }
      }
      event "Cancel": Value Change {
        n212 = event-data() -> ("NewVal"=w319:bool)  [unwired: 6 out]
        n213 = Not(x=w319) -> (.not. x?=w318:bool)
      }
      event Panel Close? {
        n214 = event-data() -> ()  [unwired: 5 out]
        n215 = event-data() -> ()  [unwired: 2 in, 1 out]
      }
      event "H_Bit 7", "H_Bit 6", "H_Bit 5", "H_Bit 4", "H_Bit 3", "H_Bit 2", "H_Bit 1", "H_Bit 0": Value Change {
        n216 = event-data() -> ("CtlRef"=w332:refnum<vi>, "NewVal"=w331:i32[])  [unwired: 5 out]
        n217 = property class="LstBox (strict)"(reference=w332) -> ("Label.Text"=w335:string)  [unwired: 1 in, 2 out]
        n218 = property class="LstBox (strict)"(reference=w332) -> ("Item Names"=w330:string[])  [unwired: 1 in, 2 out]
        n219 = local read "Message Cluster"() -> (w322:T1)
        n220 = Match Pattern(string=w335, regular expression="H_Bit ") -> (after substring=w333:string)  [unwired: 1 in, 3 out]
        n221 = for {
          tunnel: w331 -> [w337] mode=indexing
          tunnel: w330 -> [w338]
          tunnel: [w336] -> w329 mode=indexing
          n222 = Index Array(array=w338, index=w337) -> (element=w336:string)
        }
        n223 = Decimal String To Number(string=w333) -> (number=w328:i32)  [unwired: 2 in, 1 out]
        n224 = Unbundle By Name(w322) -> ("H_Bits"=w323:T2)
        n225 = Index Array(array=w323, index=w328) -> (element=w327:T6)
        n226 = Bundle By Name(cluster=w327, "Bits"=w329) -> (w326:T6)
        n227 = Replace Array Subset(array=w323, new element=w326, index=w328) -> (w325:T2)
        n228 = Bundle By Name(cluster=w322, "H_Bits"=w325) -> (w324:T1)
        n229 = local write "Message Cluster"(w324) -> ()
      }
      event "G_Bit 7", "G_Bit 6", "G_Bit 5", "G_Bit 4", "G_Bit 3", "G_Bit 2", "G_Bit 1", "G_Bit 0": Value Change {
        n230 = event-data() -> ("CtlRef"=w349:refnum<vi>, "NewVal"=w348:i32[])  [unwired: 5 out]
        n231 = property class="LstBox (strict)"(reference=w349) -> ("Label.Text"=w352:string)  [unwired: 1 in, 2 out]
        n232 = property class="LstBox (strict)"(reference=w349) -> ("Item Names"=w347:string[])  [unwired: 1 in, 2 out]
        n233 = local read "Message Cluster"() -> (w339:T1)
        n234 = Match Pattern(string=w352, regular expression="G_Bit ") -> (after substring=w350:string)  [unwired: 1 in, 3 out]
        n235 = Decimal String To Number(string=w350) -> (number=w346:i32)  [unwired: 2 in, 1 out]
        n236 = for {
          tunnel: w348 -> [w354] mode=indexing
          tunnel: w347 -> [w355]
          tunnel: [w353] -> w344 mode=indexing
          n237 = Index Array(array=w355, index=w354) -> (element=w353:string)
        }
        n238 = Unbundle By Name(w339) -> ("G_Bits"=w340:T2)
        n239 = Index Array(array=w340, index=w346) -> (element=w345:T6)
        n240 = Bundle By Name(cluster=w345, "Bits"=w344) -> (w343:T6)
        n241 = Replace Array Subset(array=w340, new element=w343, index=w346) -> (w342:T2)
        n242 = Bundle By Name(cluster=w339, "G_Bits"=w342) -> (w341:T1)
        n243 = local write "Message Cluster"(w341) -> ()
      }
      event "H_Invert 7", "H_Invert 6", "H_Invert 5", "H_Invert 4", "H_Invert 3", "H_Invert 2", "H_Invert 1", "H_Invert 0": Value Change {
        n244 = event-data() -> ("CtlRef"=w363:refnum<vi>, "NewVal"=w362:bool)  [unwired: 5 out]
        n245 = property class="Bool (strict)"(reference=w363) -> ("Label.Text"=w367:string)  [unwired: 1 in, 2 out]
        n246 = local read "Message Cluster"() -> (w356:T1)
        n247 = Match Pattern(string=w367, regular expression="H_Invert ") -> (after substring=w365:string)  [unwired: 1 in, 3 out]
        n248 = Unbundle By Name(w356) -> ("H_Bits"=w357:T2)
        n249 = Decimal String To Number(string=w365) -> (number=w364:i32)  [unwired: 2 in, 1 out]
        n250 = Index Array(array=w357, index=w364) -> (element=w361:T6)
        n251 = Bundle By Name(cluster=w361, "Invert"=w362) -> (w360:T6)
        n252 = Replace Array Subset(array=w357, new element=w360, index=w364) -> (w359:T2)
        n253 = Bundle By Name(cluster=w356, "H_Bits"=w359) -> (w358:T1)
        n254 = local write "Message Cluster"(w358) -> ()
      }
      event "G_Invert 7", "G_Invert 6", "G_Invert 5", "G_Invert 4", "G_Invert 3", "G_Invert 2", "G_Invert 1", "G_Invert 0": Value Change {
        n255 = event-data() -> ("CtlRef"=w375:refnum<vi>, "NewVal"=w374:bool)  [unwired: 5 out]
        n256 = property class="Bool (strict)"(reference=w375) -> ("Label.Text"=w379:string)  [unwired: 1 in, 2 out]
        n257 = local read "Message Cluster"() -> (w368:T1)
        n258 = Match Pattern(string=w379, regular expression="G_Invert ") -> (after substring=w377:string)  [unwired: 1 in, 3 out]
        n259 = Unbundle By Name(w368) -> ("G_Bits"=w369:T2)
        n260 = Decimal String To Number(string=w377) -> (number=w376:i32)  [unwired: 2 in, 1 out]
        n261 = Index Array(array=w369, index=w376) -> (element=w373:T6)
        n262 = Bundle By Name(cluster=w373, "Invert"=w374) -> (w372:T6)
        n263 = Replace Array Subset(array=w369, new element=w372, index=w376) -> (w371:T2)
        n264 = Bundle By Name(cluster=w368, "G_Bits"=w371) -> (w370:T1)
        n265 = local write "Message Cluster"(w370) -> ()
      }
      event "H_All 7", "H_All 6", "H_All 5", "H_All 4", "H_All 3", "H_All 2", "H_All 1", "H_All 0": Value Change {
        n266 = event-data() -> ("CtlRef"=w393:refnum<vi>, "NewVal"=w390:bool)  [unwired: 5 out]
        n267 = property class="Bool (strict)"(reference=w393) -> ("Label.Text"=w398:string)  [unwired: 1 in, 2 out]
        n268 = local read "Message Cluster"() -> (w384:T1)
        n269 = Match Pattern(string=w398, regular expression="H_All ") -> (after substring=w392:string)  [unwired: 1 in, 3 out]
        n270 = Decimal String To Number(string=w392) -> (number=w382:i32)  [unwired: 2 in, 1 out]
        n271 = Select(t=T3."Disabled and Grayed Out" ("Disabled"), s=w390, f=T3."Enabled" ("Disabled")) -> (s? t:f=w387:T3)
        n272 = local read "H Selected"() -> (w383:bool[])
        n273 = Unbundle By Name(w384) -> ("H_Bits"=w386:T2)
        n274 = Index Array(array=w383, index=w382) -> (element=w381:bool)
        n275 = Index Array(array=w386, index=w382) -> (element=w396:T6)
        n276 = case shown="False" w381 {
          tunnel: w387 -> [_ w400]
          tunnel: w382 -> [_ w399]
          frame False {
          }
          frame True {
            n277 = case shown="0, Default" w399 {
              tunnel: w400 -> [w401 w402 w403 w404 w405 w406 w407 w408]
              frame 0, Default {
                n278 = property on="H_Bit 0" class="LstBox (strict)"("DisabledEnum"=w401) -> ()  [unwired: 2 in, 2 out]
              }
              frame 1 {
                n279 = property on="H_Bit 1" class="LstBox (strict)"("DisabledEnum"=w402) -> ()  [unwired: 2 in, 2 out]
              }
              frame 2 {
                n280 = property on="H_Bit 2" class="LstBox (strict)"("DisabledEnum"=w403) -> ()  [unwired: 2 in, 2 out]
              }
              frame 3 {
                n281 = property on="H_Bit 3" class="LstBox (strict)"("DisabledEnum"=w404) -> ()  [unwired: 2 in, 2 out]
              }
              frame 4 {
                n282 = property on="H_Bit 4" class="LstBox (strict)"("DisabledEnum"=w405) -> ()  [unwired: 2 in, 2 out]
              }
              frame 5 {
                n283 = property on="H_Bit 5" class="LstBox (strict)"("DisabledEnum"=w406) -> ()  [unwired: 2 in, 2 out]
              }
              frame 6 {
                n284 = property on="H_Bit 6" class="LstBox (strict)"("DisabledEnum"=w407) -> ()  [unwired: 2 in, 2 out]
              }
              frame 7 {
                n285 = property on="H_Bit 7" class="LstBox (strict)"("DisabledEnum"=w408) -> ()  [unwired: 2 in, 2 out]
              }
            }
          }
        }
        n286 = Bundle By Name(cluster=w396, "All"=w390) -> (w395:T6)
        n287 = case shown="True" w390 {
          tunnel: w395 -> [w409 w412]
          tunnel: [w409 w411] -> w394
          tunnel: w391 -> [_ w410]
          frame False {
          }
          frame True {
            n288 = Bundle By Name(cluster=w412, "Bits"=w410) -> (w411:T6)
          }
        }
        n289 = Replace Array Subset(array=w386, new element=w394, index=w382) -> (w385:T2)
        n290 = Bundle By Name(cluster=w384, "H_Bits"=w385) -> (w380:T1)
        n291 = local write "Message Cluster"(w380) -> ()
      }
      event "G_All 7", "G_All 6", "G_All 5", "G_All 4", "G_All 3", "G_All 2", "G_All 1", "G_All 0": Value Change {
        n292 = event-data() -> ("CtlRef"=w429:refnum<vi>, "NewVal"=w424:bool)  [unwired: 5 out]
        n293 = property class="Bool (strict)"(reference=w429) -> ("Label.Text"=w431:string)  [unwired: 1 in, 2 out]
        n294 = local read "Message Cluster"() -> (w416:T1)
        n295 = Match Pattern(string=w431, regular expression="G_All ") -> (after substring=w427:string)  [unwired: 1 in, 3 out]
        n296 = local read "G Selected"() -> (w415:bool[])
        n297 = Unbundle By Name(w416) -> ("G_Bits"=w417:T2)
        n298 = Select(t=T3."Disabled and Grayed Out" ("Disabled"), s=w424, f=T3."Enabled" ("Disabled")) -> (s? t:f=w423:T3)
        n299 = Decimal String To Number(string=w427) -> (number=w414:i32)  [unwired: 2 in, 1 out]
        n300 = Index Array(array=w415, index=w414) -> (element=w413:bool)
        n301 = Index Array(array=w417, index=w414) -> (element=w422:T6)
        n302 = case shown="True" w413 {
          tunnel: w423 -> [_ w433]
          tunnel: w414 -> [_ w432]
          frame False {
          }
          frame True {
            n303 = case shown="7" w432 {
              tunnel: w433 -> [w434 w435 w436 w437 w438 w439 w440 w441]
              frame 0, Default {
                n304 = property on="G_Bit 0" class="LstBox (strict)"("DisabledEnum"=w434) -> ()  [unwired: 2 in, 2 out]
              }
              frame 1 {
                n305 = property on="G_Bit 1" class="LstBox (strict)"("DisabledEnum"=w435) -> ()  [unwired: 2 in, 2 out]
              }
              frame 2 {
                n306 = property on="G_Bit 2" class="LstBox (strict)"("DisabledEnum"=w436) -> ()  [unwired: 2 in, 2 out]
              }
              frame 3 {
                n307 = property on="G_Bit 3" class="LstBox (strict)"("DisabledEnum"=w437) -> ()  [unwired: 2 in, 2 out]
              }
              frame 4 {
                n308 = property on="G_Bit 4" class="LstBox (strict)"("DisabledEnum"=w438) -> ()  [unwired: 2 in, 2 out]
              }
              frame 5 {
                n309 = property on="G_Bit 5" class="LstBox (strict)"("DisabledEnum"=w439) -> ()  [unwired: 2 in, 2 out]
              }
              frame 6 {
                n310 = property on="G_Bit 6" class="LstBox (strict)"("DisabledEnum"=w440) -> ()  [unwired: 2 in, 2 out]
              }
              frame 7 {
                n311 = property on="G_Bit 7" class="LstBox (strict)"("DisabledEnum"=w441) -> ()  [unwired: 2 in, 2 out]
              }
            }
          }
        }
        n312 = Bundle By Name(cluster=w422, "All"=w424) -> (w421:T6)
        n313 = case shown="False" w424 {
          tunnel: w421 -> [w442 w445]
          tunnel: [w442 w444] -> w420
          tunnel: w428 -> [_ w443]
          frame False {
          }
          frame True {
            n314 = Bundle By Name(cluster=w445, "Bits"=w443) -> (w444:T6)
          }
        }
        n315 = Replace Array Subset(array=w417, new element=w420, index=w414) -> (w419:T2)
        n316 = Bundle By Name(cluster=w416, "G_Bits"=w419) -> (w418:T1)
        n317 = local write "Message Cluster"(w418) -> ()
      }
    }
  }
  "Result" <- w7
  n318 = flat-sequence {
    tunnel: w7 -> [_]
    frame #0 {
      n319 = local read "Message Cluster"() -> (→"Message Cluster Out":T1)
      n320 = control-ref of="This VI"() -> (w448:refnum<vi>)
      n321 = property class="VI"(reference=w448, "Front Panel.Title"="" ("Front Panel Window:Title")) -> ()  [unwired: 1 in, 2 out]
    }
  }
